vi "Sensor Locate.vi"() -> ()   [LabVIEW 2016]
uses:
  Classes/Controller/Camera/Machine Vision.ctl
  Drivers/Aerotech A3200/Aerotech VIs.lvlib
  Classes/Controller/Camera/Camera.lvclass
panel:
  in  "Go To Center":bool
  out "Top Left":dbl[](array[numeric])
  out "Bottom Right":dbl[](array[numeric])
  out "Top Right":dbl[](array[numeric])
  out "Bottom Left":dbl[](array[numeric])
  out "Sensor Angle":dbl
  out "XYZ Center":dbl[](array[numeric])
  in  "Calculate Center":bool
  in  "Record TR":bool
  in  "Record TL":bool
  in  "Record BR":bool
  in  "Record BL":bool
  out "Camera":dbl[](array[numeric])
  out "Image":T1(plugin-control)
  in  "Machine Vision":T2=enum."Tray Fiducials"
  in  "stop":bool
  in  "Joystick ON/OFF":bool
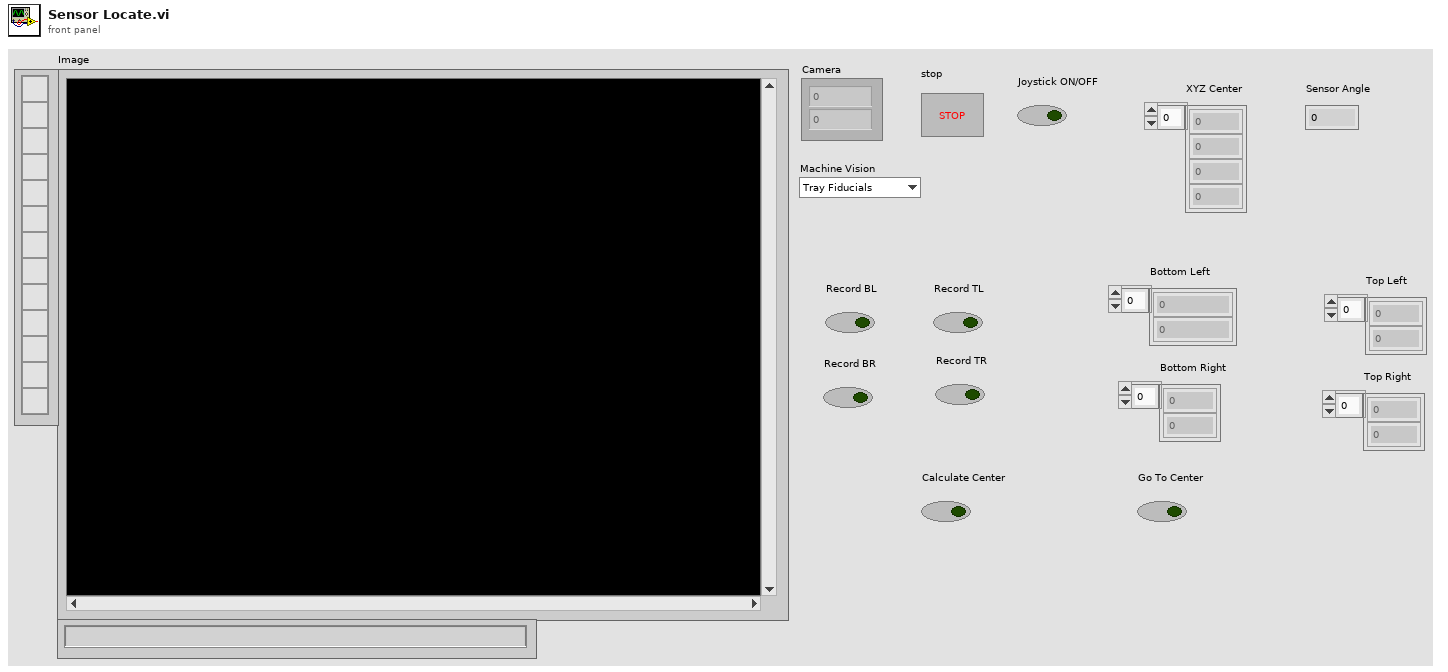
[diagram p1: front panel]
types:
  T1 = typedef "IMAQ Image.ctl" = refnum<image>
  T2 = typedef "Camera.lvclass/Machine Vision.ctl" = enum16{"None", "Tray Fiducials", "HPK Silicon", "Hexaboard", "Corner (TL, BR)", "Corner (BL, TR)"}
  T3 = typedef "Aerotech VIs.lvlib/ControllerDiagPacket.ctl" = cluster{"Number of Diag Packets":i32, "Axes":T4[], "error":errorcluster}
  T4 = typedef "Aerotech VIs.lvlib/AxisDiagPacket.ctl" = cluster{"Axis Name":string, "Analog Input 0":dbl, "Analog Input 1":dbl, "Axis Fault (num)":i32, "Axis Fault (str)":string, "Axis Fault (bits)":cluster{"AmplifierFault":bool, "AmplifierTemperatureFault":bool, "CcwEndOfTravelLimitFault":bool, "CcwSoftwareLimitFault":bool, "CommunicationLostFault":bool, "CwEndOfTravelLimitFault":bool, "CwSoftwareLimitFault":bool, "EmergencyStopFault":bool, "EncoderFault":bool, "ExternalFault":bool, "FeedbackScalingFault":bool, "GantryMisalignFault ":bool, "HallSensorFault":bool, "InPositionTimeoutFault":bool, "MarkerSearchFault":bool, "MaxVelocityCommandFault":bool, "MotorTemperatureFault":bool, "None":bool, "OverCurrentFault":bool, "PositionErrorFault":bool, "PositionFeedbackFault":bool, "PowerSupplyFault":bool, "ProbeInputFault":bool, "SafeZoneFault":bool, "VelocityErrorFault":bool, "VelocityFeedbackFault":bool, "VoltageClampFault":bool}, "Axis Status (num)":i32, "Axis Status (str)":string, "Axis Status (bits)":cluster{"BacklashActive":bool, "CalibrationEnabled1D":bool, "CalibrationEnabled2D":bool, "CommandValid":bool, "DriveAbortPending":bool, "DrivePending":bool, "Enabling":bool, "GainMappingEnabled":bool, "GantryAligned":bool, "GantryRealigning":bool, "Homed":bool, "Homing":bool, "IFOVEnabled":bool, "JogGenerating":bool, "Jogging":bool, "JoystickControl":bool, "MasterSlaveControl":bool, "MotionBlocked":bool, "MotionClamped":bool, "MoveDone":bool, "None":bool, "NotVirtual":bool, "Profiling":bool, "Stability0":bool, "Stability1":bool, "TrajectoryFiltering":bool, "WaitDone":bool}, "Current Command":sgl, "Current Error":sgl, "Current Feedback":sgl, "Digital Inputs":i32, "Digital Outputs":i32, "Drive Status":i32, "Drive Status (str)":string, "Drive Status (bits)":cluster{"AccelerationPhase":bool, "AutofocusActive":bool, "BrakeOutput":bool, "CcwEndOfTravelLimitInput":bool, "CosineEncoderError":bool, "CurrentClamp":bool, "CwEndOfTravelLimitInput":bool, "DecelerationPhase":bool, "DualLoopActive":bool, "EmergencyStopInput":bool, "Enabled":bool, "EncoderClipping":bool, "GalvoCalibrationEnabled":bool, "GalvoPowerCorrection":bool, "HallAInput":bool, "HallBInput":bool, "HallCInput":bool, "HighResolutionMode":bool, "HomeLimitInput":bool, "InPosition":bool, "InPosition2":bool, "MarkerInput":bool, "MarkerLatch":bool, "MoveActive":bool, "NoMotorSupply":bool, "None":bool, "PowerLimiting":bool, "ProgrammingFlash":bool, "ProgrammingMXH":bool, "PSOHaltLatch":bool, "ServoControl":bool, "SineEncoderError":bool}, "Position Feedback Auxiliary":dbl, "Position Command":dbl, "Position Error":dbl, "Position Feedback":dbl, "Program Position Command":dbl, "Program Position Error":dbl, "Program Position Feedback":dbl, "Velocity Command":dbl, "Velocity Error":dbl, "Velocity Feedback":dbl}
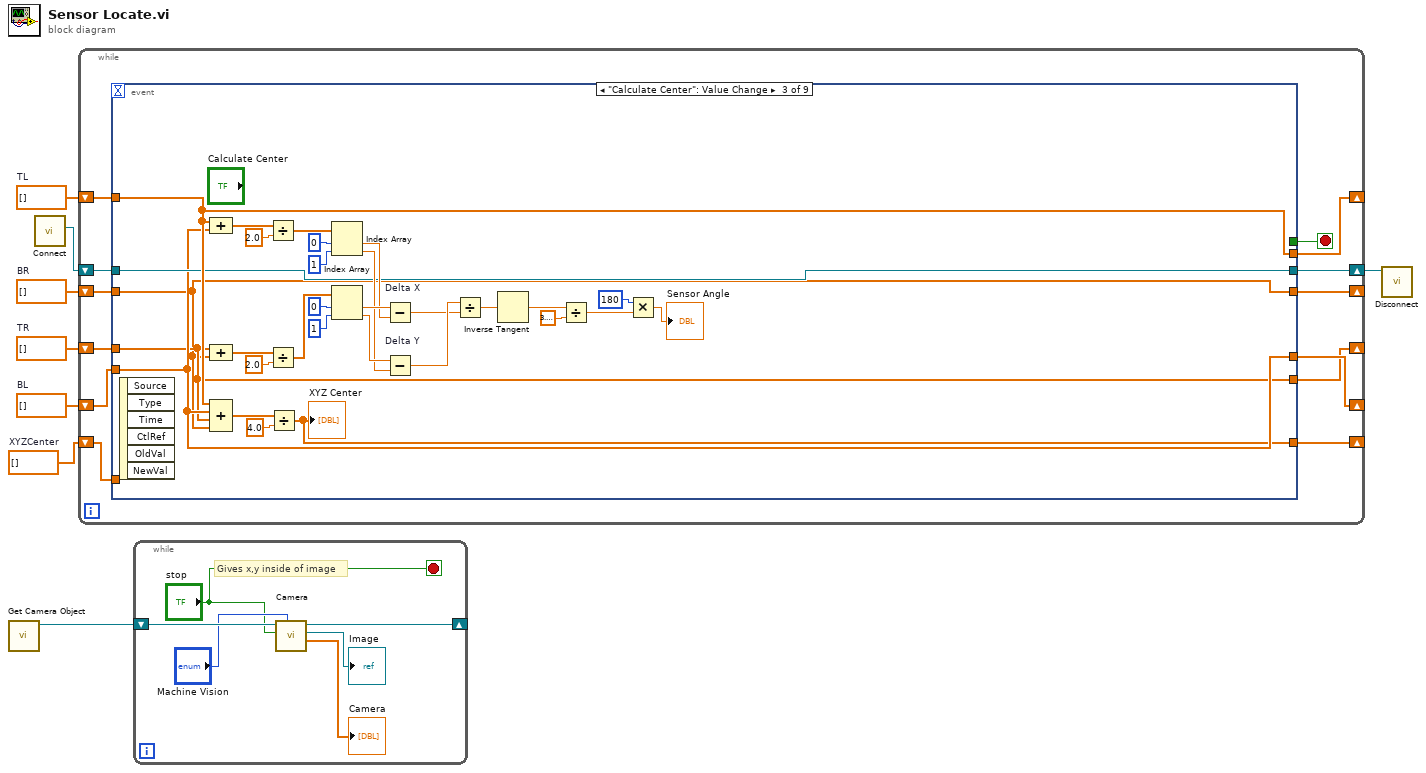
[diagram p0: block diagram]
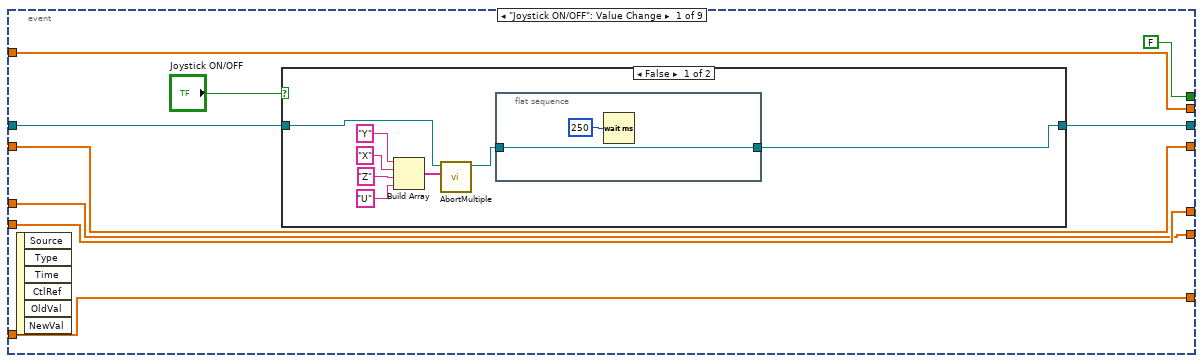
[diagram p2: hidden frame]
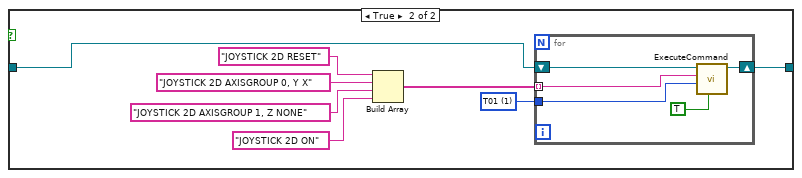
[diagram p3: hidden frame]
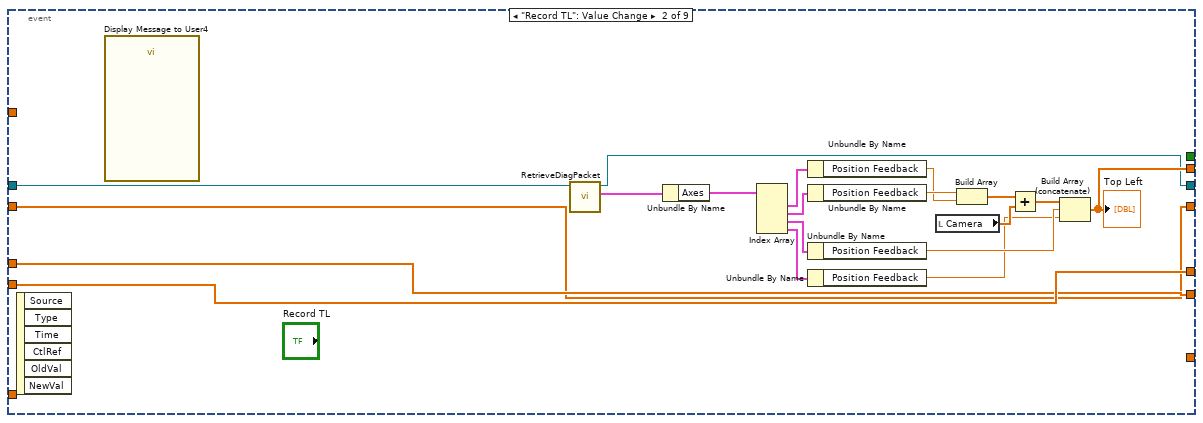
[diagram p4: hidden frame]
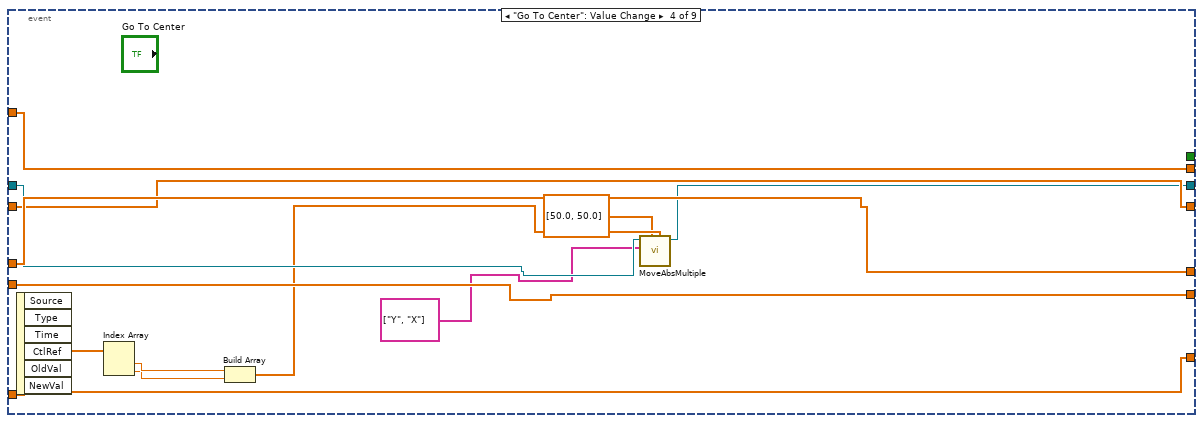
[diagram p5: hidden frame]
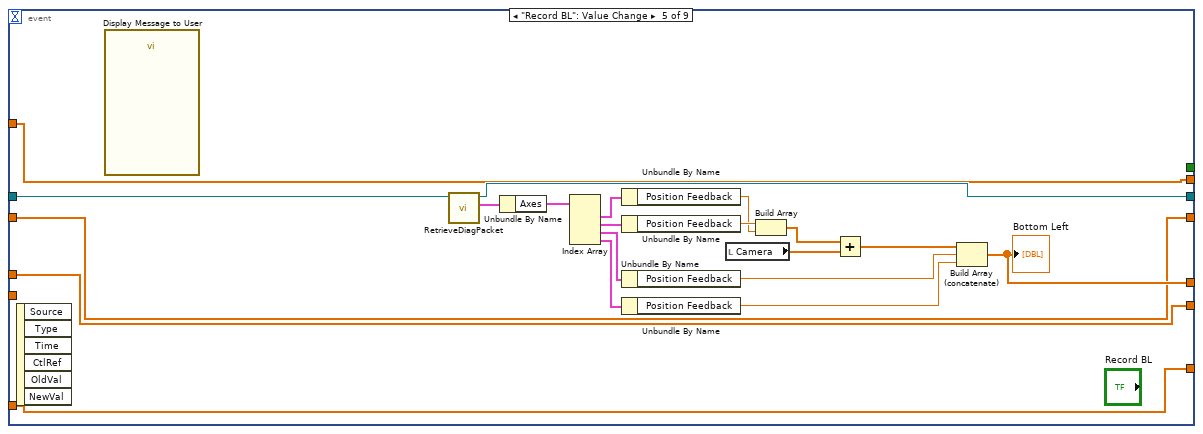
[diagram p6: hidden frame]
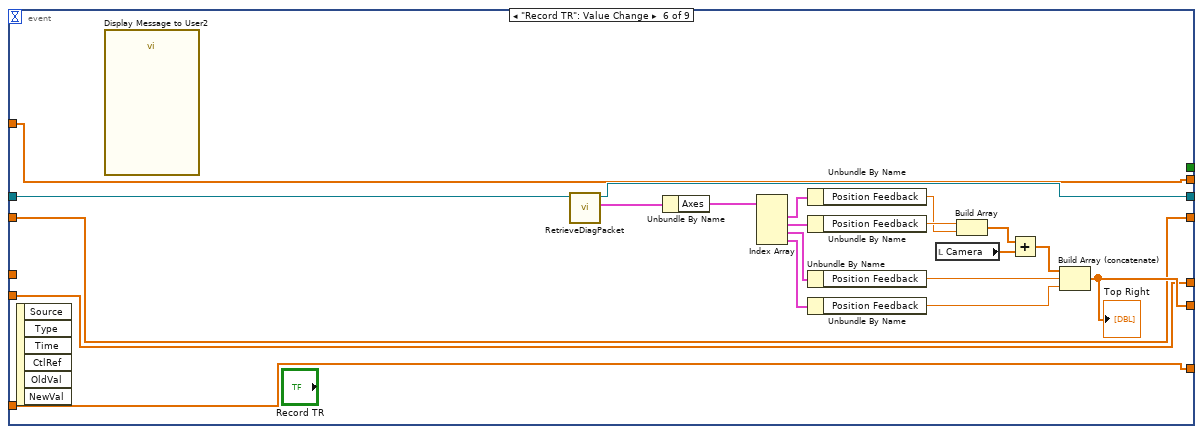
[diagram p7: hidden frame]
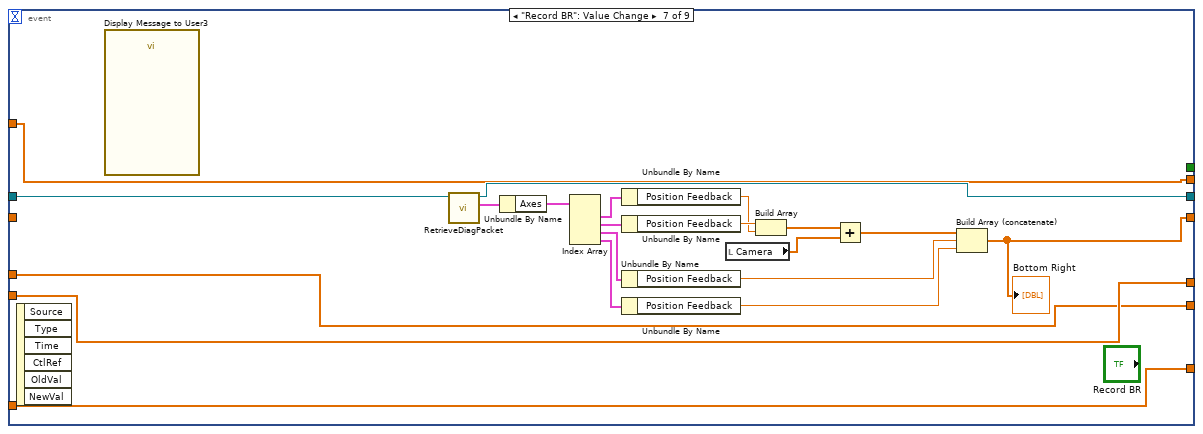
[diagram p8: hidden frame]
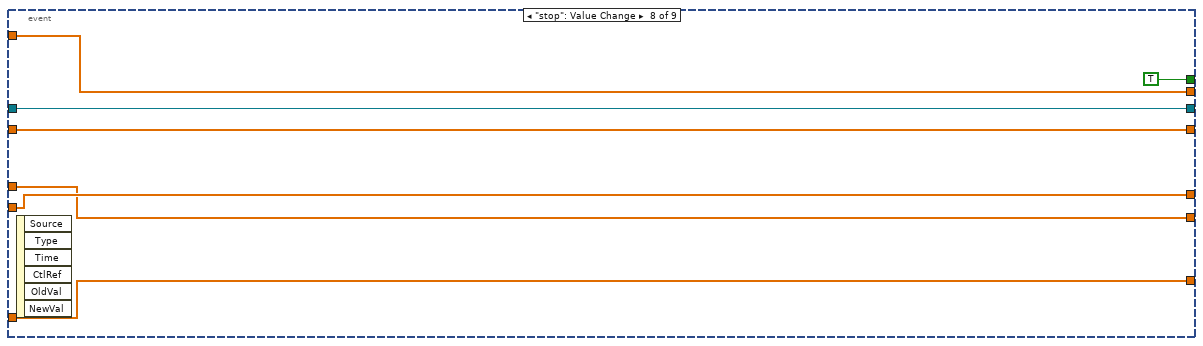
[diagram p9: hidden frame]
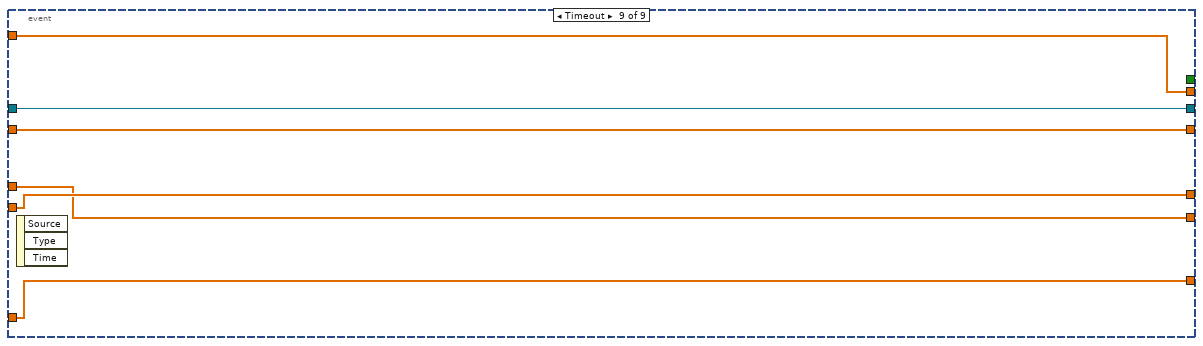
[diagram p10: hidden frame]
diagram:
  w1 = dbl[] []  # XYZCenter
  w2 = dbl[] []  # BR
  w3 = dbl[] []  # TR
  w4 = dbl[] []  # BL
  w5 = dbl[] []  # TL
  n1 = call "Get Camera Object.vi"() -> ("Camera out"=w6:refnum<class "Camera.lvclass">)  [unwired: 10 in, 1 out]
  n2 = call "Connect.vi"() -> ("controller"=w8:refnum<k24>)  [unwired: 10 in, 1 out]
  n3 = while {
    shift-right: [w20] -> w7
    shift-left: w8 -> [w21]
    shift-right: [w18] -> _
    shift-left: w5 -> [w14]
    shift-right: [w17] -> _
    shift-left: w4 -> [w13]
    shift-right: [w16] -> _
    shift-left: w3 -> [w12]
    shift-right: [w15] -> _
    shift-left: w2 -> [w11]
    shift-right: [w10] -> _
    shift-left: w1 -> [w9]
    stop <- w19 stop-if-true
    n4 = event shown="[2] \"Calculate Center\": Value Change" {
      selector: _ -> [_ _ _ _ _ _ _ _ _]
      dyn-events: _ -> [_ _ _ _ _ _ _ _ _]
      timeout: _ -> [_ _ _ _ _ _ _ _ _]
      tunnel: w21 -> [w29 w72 w83 w107 w120 w141 w161 w180 w187]
      tunnel: [w28 w54 w83 w104 w119 w140 w160 w180 w187] -> w20
      tunnel: [FALSE _ _ _ _ _ _ TRUE _] -> w19
      tunnel: [w26 w58 w84 w108 w116 w136 w158 w179 w186] -> w18
      tunnel: [w25 w57 w82 w110 w121 w137 w157 w178 w185] -> w17
      tunnel: [w24 w56 w81 w111 w117 w139 w156 w177 w184] -> w16
      tunnel: [w23 w55 w80 w109 w118 w138 w159 w176 w183] -> w15
      tunnel: w14 -> [w26 _ w84 w108 w116 w136 w158 w179 w186]
      tunnel: w13 -> [w25 w57 w82 w111 _ w137 w157 w178 w185]
      tunnel: w12 -> [w24 w56 w81 w110 w117 _ w156 w177 w184]
      tunnel: w11 -> [w23 w55 w80 w109 w118 w138 _ w176 w183]
      tunnel: [w22 _ w73 w112 w115 w135 w155 w175 w182] -> w10
      tunnel: w9 -> [w22 _ _ w112 w115 w135 w155 w175 w182]
      event "Joystick ON/OFF": Value Change {
        n5 = event-data() -> ()  [unwired: 1 in, 6 out]
        n6 = case shown="False" "Joystick ON/OFF" {
          tunnel: w29 -> [w32 w42]
          tunnel: [w31 w41] -> w28
          frame False {
            n7 = Build Array("Y" ("axis name"), "X", "Z", "U") -> (w34:string[])
            n8 = call "AbortMultiple.vi"("axis names"=w34, "controller in"=w32) -> ("controller out"=w33:refnum<k24>)  [unwired: 8 in, 1 out]
            n9 = flat-sequence {
              tunnel: w33 -> [w40]
              tunnel: [w40] -> w31
              frame #0 {
                n10 = Wait (ms)(milliseconds to wait=u32 250) -> ()  [unwired: 1 out]
              }
            }
          }
          frame True {
            w44 = 1 items=["TLibrary", "T01", "T02", "T03", "T04", "T05", "T06", "T07", "T08", "T09", "T10", "T11", "T12", "T13", "T14", "T15", "T16", "T17", "T18", "T19", "T20", "T21", "T22", "T23", "T24", "T25", "T26", "T27", "T28", "T29", "T30", "T31"] ("taskId")
            n11 = Build Array("JOYSTICK 2D RESET", "JOYSTICK 2D AXISGROUP 0, Y X", "JOYSTICK 2D AXISGROUP 1, Z NONE", "JOYSTICK 2D ON") -> (w45:string[])
            n12 = for {
              tunnel: w45 -> [w53] mode=indexing
              tunnel: w44 -> [w52]
              shift-right: [w49] -> w41
              shift-left: w42 -> [w51]
              n13 = call "ExecuteCommand.vi"("return immediately"=TRUE, "taskId"=w52, "Command Code"=w53, "controller in"=w51) -> ("controller out"=w49:refnum<k24>)  [unwired: 5 in, 2 out]
            }
          }
        }
      }
      event "Record TL": Value Change {
        n14 = event-data() -> ()  [unwired: 1 in, 6 out]
        n15 = call "Display Message to User4"() -> ()  [unwired: 10 in, 2 out]
        n16 = call "RetrieveDiagPacket.vi"("Controller In"=w72) -> ("ControllerDiagPacket"=w71:T3, "Controller Out"=w54:refnum<k24>)  [unwired: 8 in, 1 out]
        n17 = Unbundle By Name(w71) -> ("Axes"=w70:T4[])
        n18 = Index Array(array=w70) -> (element #1=w69:T4, element #2=w68:T4, element #3=w67:T4, element #4=w62:T4)  [unwired: 4 in]
        n19 = Unbundle By Name(w69) -> ("Position Feedback"=w65:dbl)
        n20 = Unbundle By Name(w68) -> ("Position Feedback"=w66:dbl)
        n21 = Unbundle By Name(w67) -> ("Position Feedback"=w60:dbl)
        n22 = Unbundle By Name(w62) -> ("Position Feedback"=w59:dbl)
        n23 = local read "Camera"() -> (w63:dbl[])
        n24 = Build Array(w66, w65) -> (w64:dbl[])
        n25 = Add(x=w64, y=w63) -> (x+y=w61:dbl[])
        n26 = Build Array (concatenate)(w61, w60, w59) -> (w58:dbl[])
        "Top Left" <- w58
      }
      event "Calculate Center": Value Change {
        n27 = event-data() -> ()  [unwired: 1 in, 6 out]
        n28 = Compound Arithmetic op=ADD(w84, w82) -> (w99:dbl[])
        n29 = Compound Arithmetic op=ADD(w81, w80) -> (w97:dbl[])
        n30 = Compound Arithmetic op=ADD(w84, w82, w81, w80) -> (w101:dbl[])
        n31 = Divide(x=w99, y=2.0) -> (x/y=w79:dbl[])
        n32 = Divide(x=w97, y=2.0) -> (x/y=w92:dbl[])
        n33 = Divide(x=w101, y=4.0) -> (x/y=w73:dbl[])
        "XYZ Center" <- w73
        n34 = Index Array(array=w79, index #1=0 ("index"), index #2=1 ("index")) -> (element #1=w90:dbl, element #2=w88:dbl)
        n35 = Index Array(array=w92, index #1=0 ("index"), index #2=1 ("index")) -> (element #1=w91:dbl, element #2=w89:dbl)
        n36 = Subtract "Delta X"(x=w91, y=w90) -> (x-y=w86:dbl)
        n37 = Subtract "Delta Y"(x=w89, y=w88) -> (x-y=w87:dbl)
        n38 = Divide(x=w87, y=w86) -> (x/y=w85:dbl)
        n39 = Inverse Tangent(1:w85) -> (0:w78:dbl)
        n40 = Divide(x=w78, y=3.141592653589793) -> (x/y=w76:dbl)
        n41 = Multiply(x=180, y=w76) -> (x*y=→"Sensor Angle":dbl)
      }
      event "Go To Center": Value Change {
        n42 = event-data() -> ()  [unwired: 1 in, 6 out]
        n43 = Index Array(array=w112) -> (element #1=w114:dbl, element #2=w113:dbl)  [unwired: 2 in]
        n44 = Build Array(w114, w113) -> (w105:dbl[])
        n45 = call "MoveAbsMultiple.vi"("positions"=w105, "speeds"=dbl[] [50.0, 50.0], "axis names"=string[] ["Y", "X"], "controller in"=w107) -> ("controller out"=w104:refnum<k24>)  [unwired: 6 in, 1 out]
      }
      event "Record BL": Value Change {
        n46 = event-data() -> ()  [unwired: 1 in, 6 out]
        n47 = call "Display Message to User"() -> ()  [unwired: 10 in, 2 out]
        n48 = call "RetrieveDiagPacket.vi"("Controller In"=w120) -> ("ControllerDiagPacket"=w134:T3, "Controller Out"=w119:refnum<k24>)  [unwired: 8 in, 1 out]
        n49 = Unbundle By Name(w134) -> ("Axes"=w133:T4[])
        n50 = Index Array(array=w133) -> (element #1=w132:T4, element #2=w131:T4, element #3=w130:T4, element #4=w126:T4)  [unwired: 4 in]
        n51 = Unbundle By Name(w132) -> ("Position Feedback"=w128:dbl)
        n52 = Unbundle By Name(w131) -> ("Position Feedback"=w129:dbl)
        n53 = Unbundle By Name(w130) -> ("Position Feedback"=w124:dbl)
        n54 = Unbundle By Name(w126) -> ("Position Feedback"=w123:dbl)
        n55 = local read "Camera"() -> (w122:dbl[])
        n56 = Build Array(w129, w128) -> (w127:dbl[])
        n57 = Add(x=w127, y=w122) -> (x+y=w125:dbl[])
        n58 = Build Array (concatenate)(w125, w124, w123) -> (w121:dbl[])
        "Bottom Left" <- w121
      }
      event "Record TR": Value Change {
        n59 = event-data() -> ()  [unwired: 1 in, 6 out]
        n60 = call "Display Message to User2"() -> ()  [unwired: 10 in, 2 out]
        n61 = call "RetrieveDiagPacket.vi"("Controller In"=w141) -> ("ControllerDiagPacket"=w154:T3, "Controller Out"=w140:refnum<k24>)  [unwired: 8 in, 1 out]
        n62 = Unbundle By Name(w154) -> ("Axes"=w153:T4[])
        n63 = Index Array(array=w153) -> (element #1=w152:T4, element #2=w151:T4, element #3=w150:T4, element #4=w145:T4)  [unwired: 4 in]
        n64 = Unbundle By Name(w152) -> ("Position Feedback"=w148:dbl)
        n65 = Unbundle By Name(w151) -> ("Position Feedback"=w149:dbl)
        n66 = Unbundle By Name(w150) -> ("Position Feedback"=w143:dbl)
        n67 = Unbundle By Name(w145) -> ("Position Feedback"=w142:dbl)
        n68 = local read "Camera"() -> (w146:dbl[])
        n69 = Build Array(w149, w148) -> (w147:dbl[])
        n70 = Add(x=w147, y=w146) -> (x+y=w144:dbl[])
        n71 = Build Array (concatenate)(w144, w143, w142) -> (w139:dbl[])
        "Top Right" <- w139
      }
      event "Record BR": Value Change {
        n72 = event-data() -> ()  [unwired: 1 in, 6 out]
        n73 = call "Display Message to User3"() -> ()  [unwired: 10 in, 2 out]
        n74 = call "RetrieveDiagPacket.vi"("Controller In"=w161) -> ("ControllerDiagPacket"=w174:T3, "Controller Out"=w160:refnum<k24>)  [unwired: 8 in, 1 out]
        n75 = Unbundle By Name(w174) -> ("Axes"=w173:T4[])
        n76 = Index Array(array=w173) -> (element #1=w172:T4, element #2=w171:T4, element #3=w170:T4, element #4=w165:T4)  [unwired: 4 in]
        n77 = Unbundle By Name(w172) -> ("Position Feedback"=w168:dbl)
        n78 = Unbundle By Name(w171) -> ("Position Feedback"=w169:dbl)
        n79 = Unbundle By Name(w170) -> ("Position Feedback"=w163:dbl)
        n80 = Unbundle By Name(w165) -> ("Position Feedback"=w162:dbl)
        n81 = local read "Camera"() -> (w166:dbl[])
        n82 = Build Array(w169, w168) -> (w167:dbl[])
        n83 = Add(x=w167, y=w166) -> (x+y=w164:dbl[])
        n84 = Build Array (concatenate)(w164, w163, w162) -> (w159:dbl[])
        "Bottom Right" <- w159
      }
      event "stop": Value Change {
        n85 = event-data() -> ()  [unwired: 1 in, 6 out]
      }
      event Timeout {
        n86 = event-data() -> ()  [unwired: 1 in, 3 out]
      }
    }
  }
  n87 = while {
    shift-right: [w191] -> _
    shift-left: w6 -> [w193]
    stop <- "stop" stop-if-true
    # "Gives x,y inside of image"
    n88 = call "Camera.vi"("Machine Vision"="Machine Vision", "Stop"="stop", "Camera in"=w193) -> ("Camera"=→"Camera":dbl[], "Image"=→"Image":T1, "Camera out"=w191:refnum<class "Camera.lvclass">)  [unwired: 5 in, 1 out]
  }
  n89 = call "Disconnect.vi"("controller"=w7) -> ()  [unwired: 10 in, 1 out]
